vi "LiCor_component_tester.vi"() -> ()   [LabVIEW 2010]
panel:
  out "data array":dbl[](array[numeric])
  out "read string":string
  out "actual bytes read":u32
  in  "string to write":string="(RS232(Poll Now))"
  in  "Component to test:":bool caption="Component to test"
  in  "stop":bool
  in  "VISA resource name":refnum<visa-resource-name>="COM1"
  # "LiCor Component Tester\n\nThis VI is a simple test of the LiCor components to make sure that they are apt to work in the master program."
  # "Poller"
  # "Setting Writer"
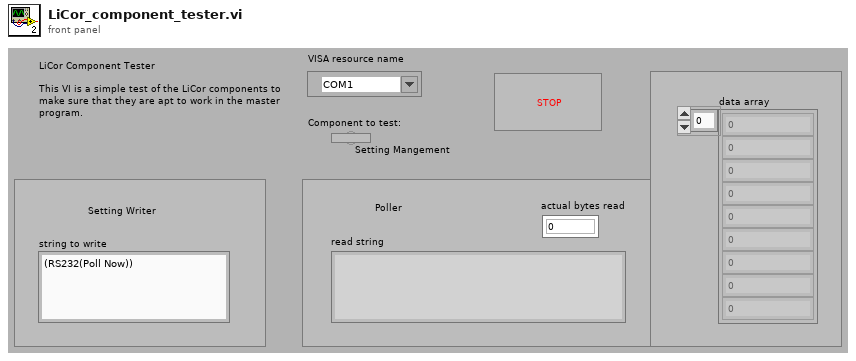
[diagram p1: front panel]
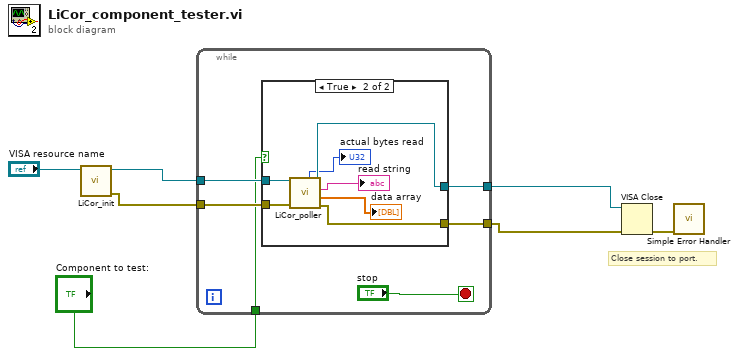
[diagram p0: block diagram]
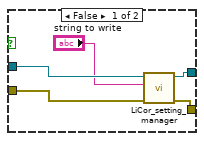
[diagram p2: hidden frame]
diagram:
  # "Close session to port."
  n1 = call "LiCor_init.vi"("VISA resource name"="VISA resource name") -> ("error out"=w4:errorcluster, "VISA out"=w5:refnum<visa-resource-name>)  [unwired: 9 in]
  n2 = while {
    tunnel: [w11] -> w3
    tunnel: [w10] -> w2
    tunnel: w5 -> [w13]
    tunnel: w4 -> [w12]
    tunnel: "Component to test:" -> [w8]
    stop <- "stop" stop-if-true
    n3 = case shown="True" w8 {
      tunnel: w13 -> [w18 w25]
      tunnel: w12 -> [w17 w24]
      tunnel: [w16 w23] -> w11
      tunnel: [w15 w22] -> w10
      frame False {
        n4 = call "LiCor_setting_manager.vi"("error in"=w17, "string to write"="string to write", "VISA session in"=w18) -> ("error out"=w15:errorcluster, "VISA session out"=w16:refnum<visa-resource-name>)  [unwired: 7 in]
      }
      frame True {
        n5 = call "LiCor_poller.vi"("error in"=w24, "VISA session in"=w25) -> ("error out"=w22:errorcluster, "data array"=→"data array":dbl[], "read string"=→"read string":string, "VISA session out"=w23:refnum<visa-resource-name>, "actual bytes read"=→"actual bytes read":u32)  [unwired: 5 in]
      }
    }
  }
  n6 = VISA Close(VISA resource name=w3, error in (no error)=w2) -> (error out=w6:errorcluster)
  n7 = call <vilib>:"Simple Error Handler.vi"("error in (no error)"=w6) -> ()  [unwired: 1 in, 8 out]
